vi "SetLedDrive(SubVI).vi"(4 "blue dac":u16, 7 "sn":string, 9 "red dac":u16) -> (3 "String":string)   [LabVIEW 2012]
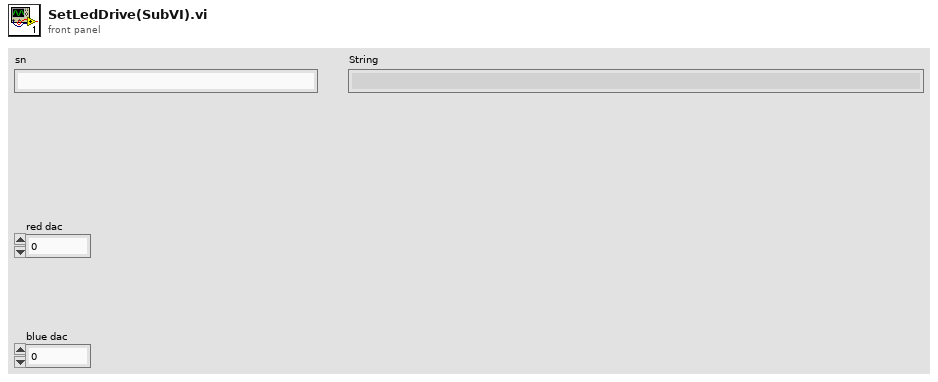
[diagram p1: front panel]
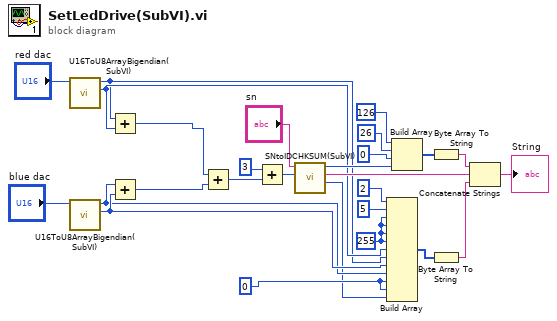
[diagram p0: block diagram]
diagram:
  w2 = 0
  w20 = u8 255
  n1 = call "U16ToU8ArrayBigendian(SubVI).vi"("int data"="red dac") -> ("low byte"=w6:u8, "high byte"=w5:u8)  [unwired: 9 in]
  n2 = call "U16ToU8ArrayBigendian(SubVI).vi"("int data"="blue dac") -> ("low byte"=w4:u8, "high byte"=w3:u8)  [unwired: 9 in]
  n3 = Add(x=w5, y=w6) -> (x+y=w7:u8)
  n4 = Add(x=w3, y=w4) -> (x+y=w8:u8)
  n5 = Add(x=w7, y=w8) -> (x+y=w12:u8)
  n6 = Add(x=u8 3, y=w12) -> (x+y=w11:u8)
  n7 = call "SNtoIDCHKSUM(SubVI).vi"("fix cheksum"=w11, "input sn"="sn") -> ("output check sum"=w1:u8, "output sn"=w24:string, "output id"=w23:u8)  [unwired: 7 in]
  n8 = Build Array(u8 2, u8 5, w20, w20, w20, w20, w6, w5, w4, w3, w2, w2, w1) -> (w16:i32[])
  n9 = Build Array(u8 126, u8 26, u8 0, w23) -> (w19:u8[])
  n10 = Byte Array To String(unsigned byte array=w19) -> (string=w22:string)
  n11 = Byte Array To String(unsigned byte array=w16) -> (string=w25:string)
  n12 = Concatenate Strings(w22, w24, w25) -> (→"String":string)
